vi "set_chart_width_4in.vi"(10 "Values to Display":dbl=400.0, 11 "Ref In":refnum<vi>) -> ()   [LabVIEW 2016]
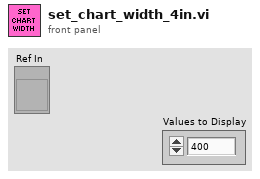
[diagram p1: front panel]
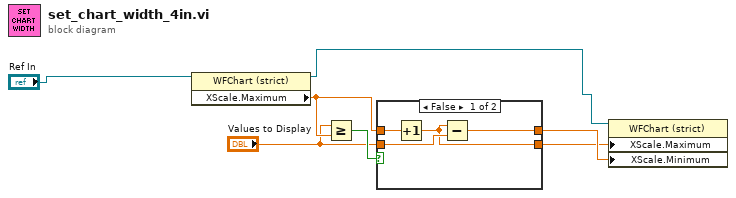
[diagram p0: block diagram]
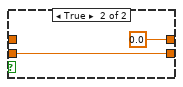
[diagram p2: hidden frame]
diagram:
  n1 = property on="Property Node" class="WFChart (strict)"(reference="Ref In") -> (reference out=w2:refnum<vi>, "XScale.Maximum"=w5:dbl)  [unwired: 1 in, 1 out]
  n2 = Greater Or Equal?(x="Values to Display", y=w5) -> (x >= y?=w4:bool)
  n3 = case shown="False" w4 {
    tunnel: "Values to Display" -> [w9 w13]
    tunnel: w5 -> [w11 _]
    tunnel: [w8 w13] -> w6
    tunnel: [w10 0.0] -> w7
    frame False {
      n4 = Increment(x=w11) -> (x+1=w8:dbl)
      n5 = Subtract(x=w8, y=w9) -> (x-y=w10:dbl)
    }
    frame True {
    }
  }
  n6 = property on="Property Node" class="WFChart (strict)"(reference=w2, "XScale.Maximum"=w6, "XScale.Minimum"=w7) -> ()  [unwired: 1 in, 2 out]
